vi "TestS.vi"(11 "Input cluster":T2) -> (3 "output cluster":T1)   [LabVIEW 2014]
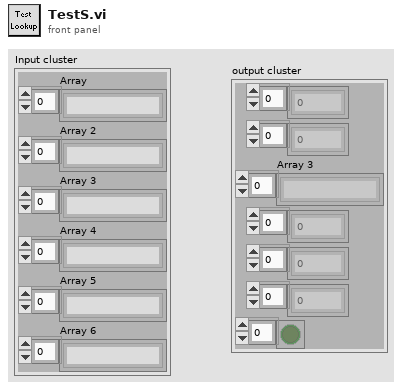
[diagram p1: front panel]
types:
  T1 = cluster{i32[], i32[], "Array 3":string[], i32[], i32[], i32[], bool[]}
  T2 = cluster{"Array":string[], "Array 2":string[], "Array 3":string[], "Array 4":string[], "Array 5":string[], "Array 6":string[]}
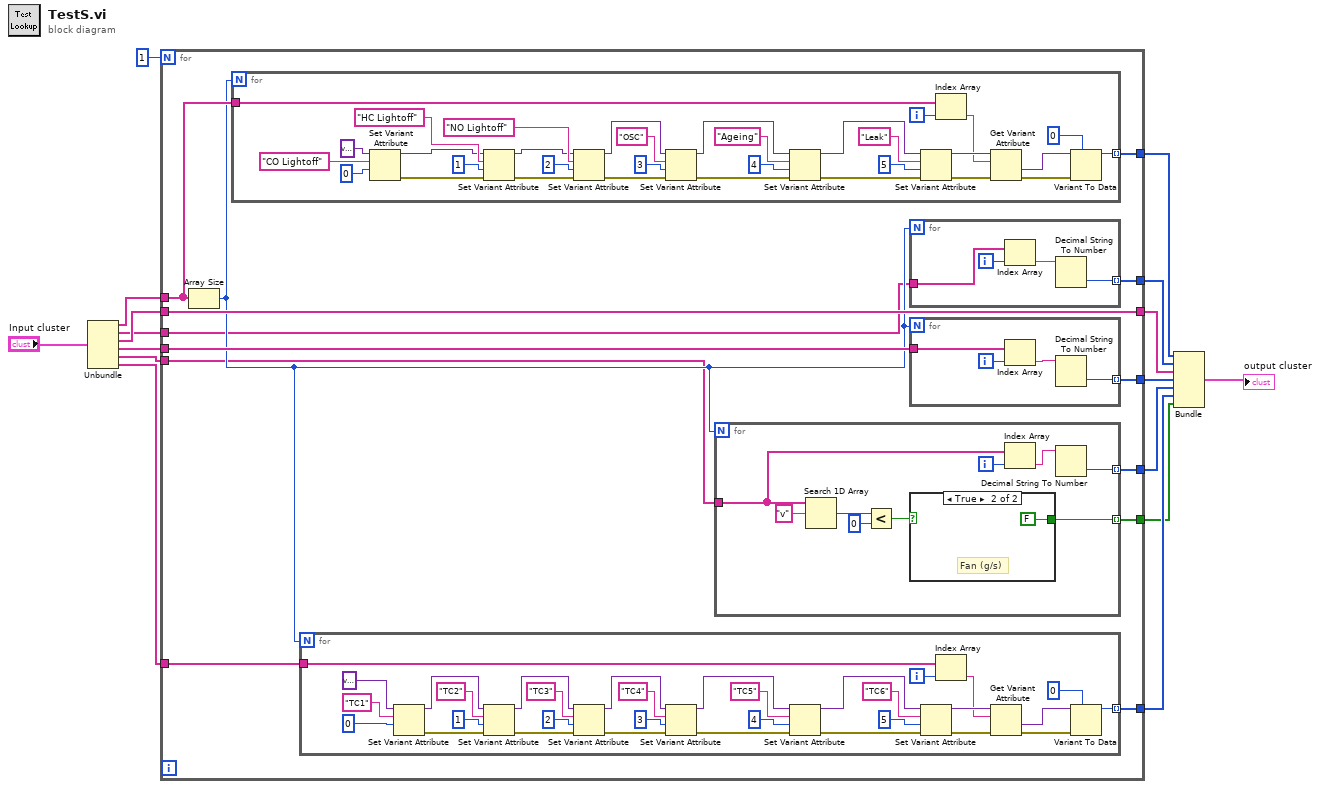
[diagram p0: block diagram]
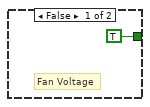
[diagram p2: hidden frame]
diagram:
  n1 = Unbundle("Input cluster") -> ("Array"=w8:string[], "Array 2"=w3:string[], "Array 3"=w7:string[], "Array 4"=w6:string[], "Array 5"=w5:string[], "Array 6"=w4:string[])
  n2 = for {
    N: 1 -> [_]
    tunnel: [w29] -> w10
    tunnel: [w28] -> w11
    tunnel: [w27] -> w12
    tunnel: [w26] -> w14
    tunnel: [w25] -> w15
    tunnel: w6 -> [w24]
    tunnel: w5 -> [w18]
    tunnel: w4 -> [w23]
    tunnel: w8 -> [w22]
    tunnel: w7 -> [w21]
    tunnel: [w21] -> w13
    tunnel: w3 -> [w19]
    tunnel: [w17] -> w2
    n3 = Array Size(array=w22) -> (size(s)=w20:i32)
    n4 = for {
      N: w20 -> [_]
      tunnel: [w85] -> w25 mode=indexing
      tunnel: w22 -> [w82]
      i -> [w83]
      n5 = Set Variant Attribute(Variant=variant, name="CO Lightoff", value=0) -> (Variant out=w89:variant, error out=w90:errorcluster)  [unwired: 1 in, 1 out]
      n6 = Set Variant Attribute(Variant=w89, name="HC Lightoff", value=1, error in=w90) -> (Variant out=w93:variant, error out=w94:errorcluster)  [unwired: 1 out]
      n7 = Set Variant Attribute(Variant=w93, name="NO Lightoff", value=2, error in=w94) -> (Variant out=w101:variant, error out=w102:errorcluster)  [unwired: 1 out]
      n8 = Set Variant Attribute(Variant=w101, name="OSC", value=3 ("index"), error in=w102) -> (Variant out=w103:variant, error out=w104:errorcluster)  [unwired: 1 out]
      n9 = Set Variant Attribute(Variant=w103, name="Ageing", value=4 ("index"), error in=w104) -> (Variant out=w107:variant, error out=w108:errorcluster)  [unwired: 1 out]
      n10 = Set Variant Attribute(Variant=w107, name="Leak", value=5 ("index"), error in=w108) -> (Variant out=w111:variant, error out=w112:errorcluster)  [unwired: 1 out]
      n11 = Index Array(array=w82, index=w83) -> (element=w81:string)
      n12 = Get Variant Attribute(Variant=w111, name=w81, error in=w112) -> (value=w84:variant, error out=w97:errorcluster)  [unwired: 1 in, 2 out]
      n13 = Variant To Data(error in=w97, type=0, Variant=w84) -> (data=w85:i32)  [unwired: 1 out]
    }
    n14 = for {
      N: w20 -> [_]
      tunnel: w23 -> [w61]
      tunnel: [w31] -> w29 mode=indexing
      i -> [w30]
      n15 = Set Variant Attribute(Variant=variant, name="TC1", value=0) -> (Variant out=w49:variant, error out=w50:errorcluster)  [unwired: 1 in, 1 out]
      n16 = Set Variant Attribute(Variant=w49, name="TC2", value=1, error in=w50) -> (Variant out=w53:variant, error out=w54:errorcluster)  [unwired: 1 out]
      n17 = Set Variant Attribute(Variant=w53, name="TC3", value=2, error in=w54) -> (Variant out=w59:variant, error out=w60:errorcluster)  [unwired: 1 out]
      n18 = Set Variant Attribute(Variant=w59, name="TC4", value=3 ("index"), error in=w60) -> (Variant out=w39:variant, error out=w38:errorcluster)  [unwired: 1 out]
      n19 = Set Variant Attribute(Variant=w39, name="TC5", value=4 ("index"), error in=w38) -> (Variant out=w40:variant, error out=w36:errorcluster)  [unwired: 1 out]
      n20 = Set Variant Attribute(Variant=w40, name="TC6", value=5 ("index"), error in=w36) -> (Variant out=w34:variant, error out=w35:errorcluster)  [unwired: 1 out]
      n21 = Index Array(array=w61, index=w30) -> (element=w33:string)
      n22 = Get Variant Attribute(Variant=w34, name=w33, error in=w35) -> (value=w32:variant, error out=w44:errorcluster)  [unwired: 1 in, 2 out]
      n23 = Variant To Data(error in=w44, type=0 ("index"), Variant=w32) -> (data=w31:i32)  [unwired: 1 out]
    }
    n24 = for {
      N: w20 -> [_]
      tunnel: w18 -> [w67]
      tunnel: [w68] -> w28 mode=indexing
      tunnel: [w62] -> w17 mode=indexing
      i -> [w70]
      n25 = Search 1D Array(1D array=w67, element="v") -> (index of element=w64:i32)  [unwired: 1 in]
      n26 = Less?(x=w64, y=0) -> (x < y?=w63:bool)
      n27 = case shown="True" w63 {
        tunnel: [TRUE FALSE] -> w62
        frame False {
          # "Fan Voltage"
        }
        frame True {
          # "Fan (g/s)"
        }
      }
      n28 = Index Array(array=w67, index=w70) -> (element=w69:string)
      n29 = Decimal String To Number(string=w69) -> (number=w68:i32)  [unwired: 2 in, 1 out]
    }
    n30 = for {
      N: w20 -> [_]
      tunnel: w19 -> [w78]
      tunnel: [w77] -> w26 mode=indexing
      i -> [w80]
      n31 = Index Array(array=w78, index=w80) -> (element=w79:string)
      n32 = Decimal String To Number(string=w79) -> (number=w77:i32)  [unwired: 2 in, 1 out]
    }
    n33 = for {
      N: w20 -> [_]
      tunnel: w24 -> [w74]
      tunnel: [w73] -> w27 mode=indexing
      i -> [w76]
      n34 = Index Array(array=w74, index=w76) -> (element=w75:string)
      n35 = Decimal String To Number(string=w75) -> (number=w73:i32)  [unwired: 2 in, 1 out]
    }
  }
  n36 = Bundle(w15, w14, "Array 3"=w13, w12, w11, w10, w2) -> (→"output cluster":T1)  [unwired: 1 in]
